vi "Read Initialization.vi"(8 "error in (no error)":errorcluster, 11 "Interface in":refnum<class "Interface.lvclass">) -> (0 "error out":errorcluster, 2 "Initialization":T1, 3 "Interface out":refnum<class "Interface.lvclass">)   [LabVIEW 2018]
uses:
  Interface.lvclass
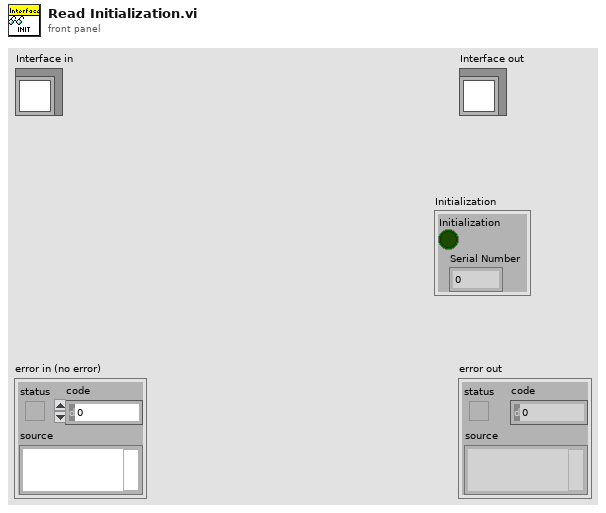
[diagram p1: front panel]
types:
  T1 = cluster{"Initialization":bool, "Serial Number":u16}
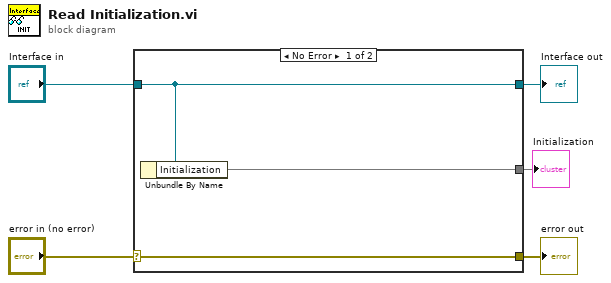
[diagram p0: block diagram]
diagram:
  n1 = case shown="No Error" "error in (no error)" {
    selector: "error in (no error)" -> [w8 w9]
    tunnel: [w8 w9] -> w4
    tunnel: [w7 w10] -> w2
    tunnel: "Interface in" -> [w7 w10]
    tunnel: [w6 _] -> w1
    frame No Error {
      n2 = Unbundle By Name(w7) -> ("Initialization"=w6)
    }
    frame Error {
    }
  }
  "error out" <- w4
  "Interface out" <- w2
  "Initialization" <- w1
